vi "Toggle.vi"(1 "Boolean":bool) -> (0 "Boolean 2":bool)   [LabVIEW 2012]
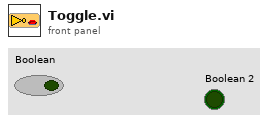
[diagram p1: front panel]
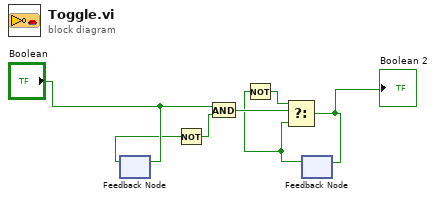
[diagram p0: block diagram]
diagram:
  n1 = feedback #1() -> (w5:bool)  [unwired: 1 in]
  n2 = feedback-in #1("Boolean") -> ()
  n3 = Not(x=w5) -> (.not. x?=w7:bool)
  n4 = And(x="Boolean", y=w7) -> (x .and. y?=w4:bool)
  n5 = feedback #2() -> (w1:bool)  [unwired: 1 in]
  n6 = Not(x=w1) -> (.not. x?=w2:bool)
  n7 = Select(t=w2, s=w4, f=w1) -> (s? t:f=w3:bool)
  "Boolean 2" <- w3
  n8 = feedback-in #2(w3) -> ()
